vi "AMZ_S3_APIHLP_Parse GET Object Request Parameters.vi"(7 "GET Object Request Parameters":T2, 8 "error in (no error)":errorcluster, 11 "HTTP Headers in":T1[](array[typedef])) -> (0 "error out":errorcluster, 3 "HTTP Headers":T1[](array[typedef]))   [LabVIEW 2015, in "LV Interface for Amazon S3.lvlib"]
uses:
  LV Interface for Amazon S3.lvlib
  Typedefs/AMZ_S3_API_GET Object Request Parameters.ctl
  Typedefs/AMZ_S3_API_GET Request Range.ctl
  Typedefs/AMZ_S3_HTTP Header-Value pair.ctl
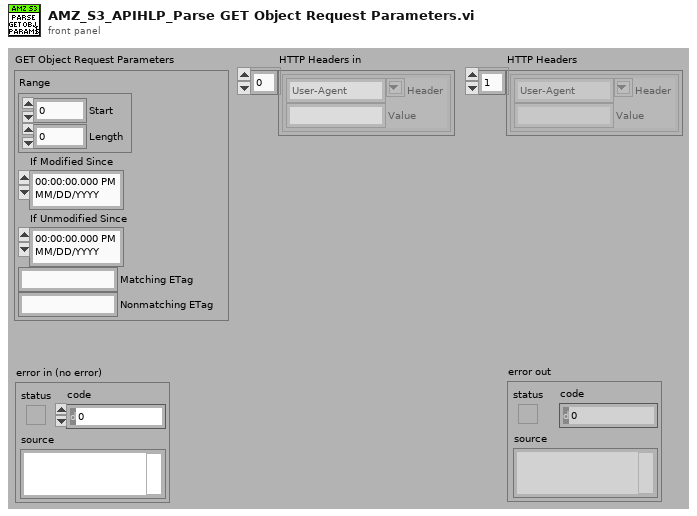
[diagram p1: front panel]
types:
  T1 = typedef "LV Interface for Amazon S3.lvlib/AMZ_S3_HTTP Header-Value pair.ctl" = cluster{"Header":string, "Value":string}
  T2 = typedef "LV Interface for Amazon S3.lvlib/AMZ_S3_API_GET Object Request Parameters.ctl" = cluster{"Range":T3, "If Modified Since":timestamp, "If Unmodified Since":timestamp, "Matching ETag":string, "Nonmatching ETag":string}
  T3 = typedef "LV Interface for Amazon S3.lvlib/AMZ_S3_API_GET Request Range.ctl" = cluster{"Start":i64, "Length":i64}
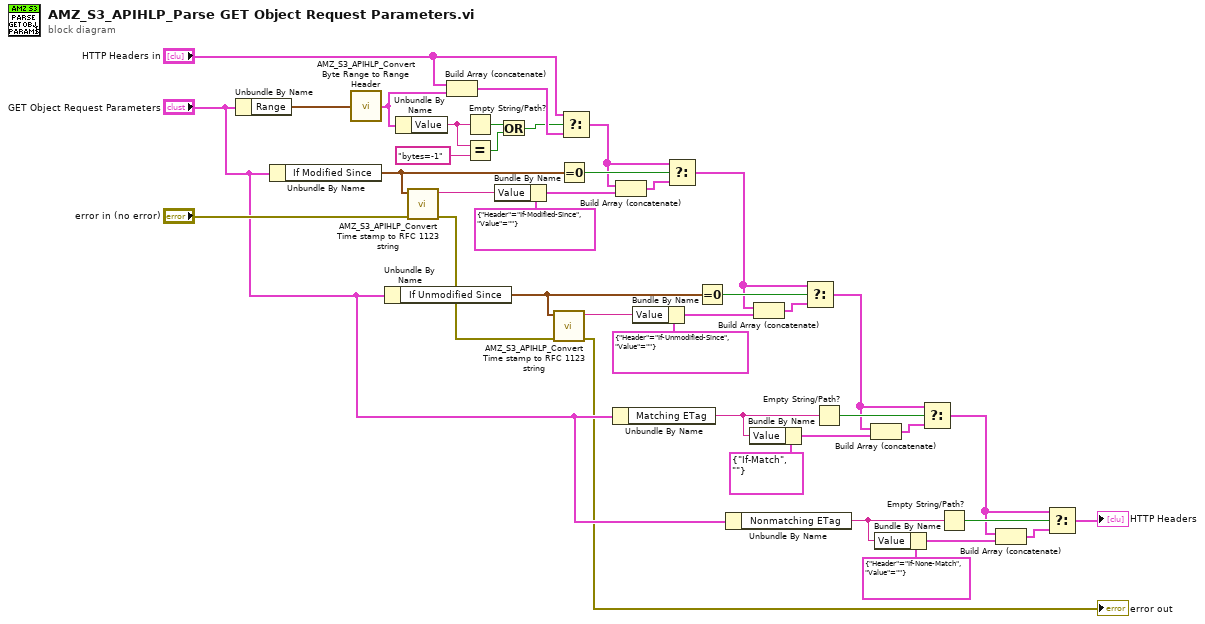
[diagram p0: block diagram]
diagram:
  n1 = Unbundle By Name("GET Object Request Parameters") -> ("Range"=w40:T3)
  n2 = Unbundle By Name("GET Object Request Parameters") -> ("If Modified Since"=w29:timestamp)
  n3 = call "AMZ_S3_APIHLP_Convert Byte Range to Range Header.vi"("Range"=w40) -> ("HTTP Header-Value pair"=w39:T1)  [unwired: 4 in]
  n4 = Unbundle By Name("GET Object Request Parameters") -> ("If Unmodified Since"=w28:timestamp)
  n5 = Unbundle By Name(w39) -> ("Value"=w5:string)
  n6 = call "AMZ_S3_APIHLP_Convert Time stamp to RFC 1123 string.vi"("error in"="error in (no error)", "time stamp"=w29) -> ("error out"=w22:errorcluster, "DateTime String (RFC-1123)"=w33:string)  [unwired: 8 in]
  n7 = Build Array (concatenate)("HTTP Headers in", w39) -> (w38:T1[])
  n8 = Empty String/Path?(string/path=w5) -> (empty?=w2:bool)
  n9 = Equal?(x=w5, y="bytes=-1") -> (x = y?=w3:bool)
  n10 = Bundle By Name(cluster=T1 {"Header"="If-Modified-Since", "Value"=""} ("HTTP Header-Value pair"), "Value"=w33) -> (w31:T1)
  n11 = Or(x=w2, y=w3) -> (x .or. y?=w1:bool)
  n12 = call "AMZ_S3_APIHLP_Convert Time stamp to RFC 1123 string.vi"("error in"=w22, "time stamp"=w28) -> ("error out"=→"error out":errorcluster, "DateTime String (RFC-1123)"=w25:string)  [unwired: 8 in]
  n13 = Equal To 0?(x=w29) -> (x = 0?=w36:bool)
  n14 = Select(t="HTTP Headers in", s=w1, f=w38) -> (s? t:f=w32:T1[])
  n15 = Unbundle By Name("GET Object Request Parameters") -> ("Matching ETag"=w15:string)
  n16 = Build Array (concatenate)(w32, w31) -> (w30:T1[])
  n17 = Bundle By Name(cluster=T1 {"Header"="If-Unmodified-Since", "Value"=""} ("HTTP Header-Value pair"), "Value"=w25) -> (w26:T1)
  n18 = Select(t=w32, s=w36, f=w30) -> (s? t:f=w21:T1[])
  n19 = Equal To 0?(x=w28) -> (x = 0?=w23:bool)
  n20 = Unbundle By Name("GET Object Request Parameters") -> ("Nonmatching ETag"=w14:string)
  n21 = Bundle By Name(cluster=T1 {"Header"="If-Match", "Value"=""} ("HTTP Header-Value pair"), "Value"=w15) -> (w18:T1)
  n22 = Build Array (concatenate)(w21, w26) -> (w27:T1[])
  n23 = Select(t=w21, s=w23, f=w27) -> (s? t:f=w16:T1[])
  n24 = Empty String/Path?(string/path=w15) -> (empty?=w20:bool)
  n25 = Build Array (concatenate)(w16, w18) -> (w17:T1[])
  n26 = Bundle By Name(cluster=T1 {"Header"="If-None-Match", "Value"=""} ("HTTP Header-Value pair"), "Value"=w14) -> (w12:T1)
  n27 = Select(t=w16, s=w20, f=w17) -> (s? t:f=w9:T1[])
  n28 = Empty String/Path?(string/path=w14) -> (empty?=w10:bool)
  n29 = Build Array (concatenate)(w9, w12) -> (w13:T1[])
  n30 = Select(t=w9, s=w10, f=w13) -> (s? t:f=→"HTTP Headers":T1[])
